vi "Digital_Bridge_3_kart.vi"() -> ()   [LabVIEW 2014] (continued)
            # "Bu bölüm, iterasyona (tekrarlamalı işleme) bağlı olarak Reserve ayarının maksimumda mı yoksa minimumda mı olacağını belirler. Aynı zamanda, ölçüm sürecinin başlangıcında kullanılacak olan sensitivity  değerleri de bu bölümde ayarlanır. Bu ayarlar, ölçüm sırasında cihazın hassasiyetini ve çalışma aralığını doğru şekilde belirlemek için gereklidir."
            # "ana denge"
            n1007 = case shown="True" "Ana denge Switch" {
              frame False {
              }
              frame True {
                # "Ana denge switch ayarlanıyor ve global x ve y set ediliyor"
                n1008 = flat-sequence {
                  frame #0 {
                    n1009 = local read "iterasyon AD"() -> (w4688:dbl)
                    n1010 = Equal?(x=w4688, y=0.0) -> (x = y?=w4689:bool)
                    n1011 = case shown="True" w4689 {
                      frame False {
                      }
                      frame True {
                        n1012 = local read "1 or 10"() -> (w4691:i32)
                        n1013 = case shown="1" w4691 {
                          frame 0, Default {
                          }
                          frame 1 {
                            n1014 = local write "iterasyon AD"(1.0 ("iterasyon WAGNER")) -> ()
                          }
                        }
                      }
                    }
                  }
                  frame #1 {
                    n1015 = local read "iterasyon AD"() -> (w4693:dbl)
                    n1016 = local read "1 or 10"() -> (w4697:i32)
                    n1017 = Equal?(x=w4697, y=1) -> (x = y?=w4698:bool)
                    n1018 = Greater?(x=w4693, y=0.0) -> (0:w4695:bool)
                    n1019 = Or(x=w4695, y=w4698) -> (x .or. y?=w4694:bool)
                    n1020 = case shown="True" w4694 {
                      frame False {
                        n1021 = local read "Reserve AD"() -> (w4701:u16)
                        n1022 = case shown="0, Default" w4701 {
                          tunnel: ["0" ("Reserve(MAX-MIN)") "1" ("Reserve(MAX-MIN)") "2" ("Reserve(MAX-MIN)")] -> w4700
                          frame 0, Default {
                          }
                          frame 1 {
                          }
                          frame 2 {
                          }
                        }
                        n1023 = local read "GPIB In"() -> (w4702:refnum<visa-resource-name>)
                        n1024 = call "Reserve.vi"("Reserve(MAX-MIN)"=w4700, "VISA resource name"=w4702) -> ()  [unwired: 8 in, 2 out]
                      }
                      frame True {
                        n1025 = local read "GPIB In"() -> (w4707:refnum<visa-resource-name>)
                        n1026 = call "Reserve.vi"("Reserve(MAX-MIN)"="2", "VISA resource name"=w4707) -> ()  [unwired: 8 in, 2 out]
                      }
                    }
                  }
                  frame #2 {
                    n1027 = Wait (ms)(milliseconds to wait=u32 500) -> ()  [unwired: 1 out]
                  }
                  frame #3 {
                    w4710 = u16 1 items=["Wagner", "Ground"] ("Switch")
                    w4711 = u16 1 items=["Open All", "Ana Denge", "10R", "1R"] ("Ring")
                    n1028 = call "mux1.vi"("Ring"=w4711) -> ("error out"=w4712:errorcluster)  [unwired: 9 in]
                    n1029 = property on="Tab Control" class="TabCtl (strict)"("Value"=T4."Ana Denge" ("Tab Control")) -> ()  [unwired: 2 in, 2 out]
                    n1030 = call "mux2.vi"("Switch"=w4710, "error in (no error)"=w4712) -> ()  [unwired: 6 in, 1 out]
                  }
                  frame #4 {
                    n1031 = Wait (ms)(milliseconds to wait=u32 1000) -> ()  [unwired: 1 out]
                  }
                  frame #5 {
                    n1032 = local read "1 or 10"() -> (w4717:i32)
                    n1033 = local read "İterasyon X"() -> (w4720:dbl)
                    n1034 = Equal?(x=w4717, y=1) -> (x = y?=w4716:bool)
                    n1035 = Greater?(x=w4720, y=0.0) -> (0:w4715:bool)
                    n1036 = Or(x=w4715, y=w4716) -> (x .or. y?=w4714:bool)
                    n1037 = case shown="False" w4714 {
                      frame False {
                        n1038 = local read "Y Range AD"() -> (w4721:dbl)
                        n1039 = local read "X Range AD"() -> (w4722:dbl)
                        n1040 = global write "show_sensitivity.vi" "show sensitivity (ana denge  x)"(w4722) -> ()
                        n1041 = global write "show_sensitivity.vi" "show sensitivity (ana denge  y)"(w4721) -> ()
                      }
                      frame True {
                        w4723 = 10.0 ("Max. Hassasiyet")
                        n1042 = global write "show_sensitivity.vi" "show sensitivity (ana denge  x)"(w4723) -> ()
                        n1043 = global write "show_sensitivity.vi" "show sensitivity (ana denge  y)"(w4723) -> ()
                      }
                    }
                  }
                  frame #6 {
                    n1044 = local write "Ana denge Switch"(FALSE ("wagner switch")) -> ()
                    n1045 = local write "Start AD X"(TRUE ("START WAGNER")) -> ()
                  }
                }
              }
            }
            n1046 = case shown="True" "Start AD X" {
              frame False {
              }
              frame True {
                n1047 = flat-sequence {
                  frame #0 {
                    w4665 = u16 0 items=["A", "A-B"] ("Input Source (0: A)")
                    n1048 = local read "frekans index"() -> (w4660:dbl)
                    n1049 = local read "Frekanslar"() -> (w4661:dbl[])
                    n1050 = local read "Direnc 1 - Direnc 2"() -> (w4662:u32)
                    n1051 = local read "AD F/P Array"() -> (w4663:dbl[][])
                    n1052 = Index Array(array=w4661, index=w4660) -> (element=w4659:dbl)
                    n1053 = call "get_phase_element.vi"("index r"=w4662, "hz"=w4659, "Array"=w4663) -> ("element"=w4655:dbl)  [unwired: 8 in]
                    n1054 = Number To Fractional String(number=w4655) -> (F-format string=w4658:string)  [unwired: 3 in]
                    n1055 = local read "GPIB In"() -> (w4664:refnum<visa-resource-name>)
                    n1056 = Search and Replace String(input string=w4658, search string=",", replace string="." ("replace string (\"\")")) -> (result string=w4654:string)  [unwired: 5 in, 3 out]
                    n1057 = call "reference phase.vi"("Reference Phase (0.000 degrees)"=w4654, "VISA resource name"=w4664) -> ("error out"=w4666:errorcluster, "VISA resource name out"=w4667:refnum<visa-resource-name>)  [unwired: 8 in]
                    n1058 = call "input source.vi"("error in (no error)"=w4666, "Input Source (0: A)"=w4665, "VISA resource name"=w4667) -> ()  [unwired: 7 in, 2 out]
                  }
                  frame #1 {
                    n1059 = local read "İterasyon X"() -> (w4678:dbl)
                    n1060 = local read "1 or 10"() -> (w4682:i32)
                    n1061 = local read "frekans index"() -> (w4676:dbl)
                    n1062 = local read "control hz array"() -> (w4673:dbl[][])
                    n1063 = Greater?(x=w4678, y=0.0) -> (0:w4679:bool)
                    n1064 = call "change2d.vi"("reset(default false)"=FALSE, "index (col)"=w4676, "index (row)"=2, "read/write(T/F)"=TRUE, "2D Array"=w4673) -> ("result count"=w4671:dbl)  [unwired: 5 in, 1 out]
                    n1065 = Equal?(x=w4682, y=1) -> (x = y?=w4680:bool)
                    n1066 = local read "set"() -> (w4670:u16)
                    n1067 = Or(x=w4679, y=w4680) -> (x .or. y?=w4672:bool)
                    n1068 = Equal?(x=w4671, y=w4670) -> (x = y?=w4669:bool)
                    n1069 = Or(x=w4672, y=w4669) -> (x .or. y?=w4668:bool)
                    n1070 = case shown="True" w4668 {
                      frame False {
                        n1071 = local write "auto phase AD"(TRUE ("auto phase 10R")) -> ()
                        n1072 = local write "Start AD X"(FALSE ("auto phase 10R")) -> ()
                      }
                      frame True {
                        n1073 = local write "Contiune AD"(TRUE) -> ()
                        n1074 = local write "Start AD X"(FALSE ("START WAGNER")) -> ()
                      }
                    }
                  }
                }
              }
            }
            n1075 = case shown="True" "RESET SENS X" {
              frame False {
              }
              frame True {
                n1076 = local read "count meas"() -> (w4779:u16)
                n1077 = local read "iterasyon AD"() -> (w4777:dbl)
                n1078 = Greater?(x=w4779, y=u16 8) -> (0:w4775:bool)
                n1079 = Greater?(x=w4777, y=5.0) -> (0:w4774:bool)
                n1080 = Or(x=w4775, y=w4774) -> (x .or. y?=w4773:bool)
                n1081 = case shown="True" w4773 {
                  frame False {
                    n1082 = flat-sequence {
                      frame #0 {
                        n1083 = global read "show_sensitivity.vi" "show sensitivity (ana denge  x)"() -> (w4780:dbl)
                        n1084 = local read "GPIB In"() -> (w4781:refnum<visa-resource-name>)
                        n1085 = call "get_sensitivity.vi"("input 1"=w4780, "SR850 GPIB In"=w4781) -> ()  [unwired: 8 in, 2 out]
                      }
                      frame #1 {
                        n1086 = Wait (ms)(milliseconds to wait=u32 500) -> ()  [unwired: 1 out]
                      }
                      frame #2 {
                        n1087 = local write "RESET SENS X"(FALSE ("RESET SENS X")) -> ()
                        n1088 = local write "START X"(TRUE ("START X 4")) -> ()
                      }
                    }
                  }
                  frame True {
                    n1089 = local read "iterasyon AD"() -> (w4786:dbl)
                    n1090 = Greater?(x=w4786, y=5.0) -> (0:w4785:bool)
                    n1091 = case shown="False" w4785 {
                      frame False {
                        n1092 = flat-sequence {
                          frame #0 {
                            n1093 = local write "count meas"(u16 9 ("count meas")) -> ()
                            n1094 = local write "RESET SENS X"(FALSE ("Start 10R X")) -> ()
                            n1095 = local write "İterasyon X"(0.0 ("İterasyon X")) -> ()
                          }
                          frame #1 {
                            n1096 = local write "reset values"(TRUE ("Start 10R X")) -> ()
                            n1097 = local write "error"(TRUE ("Start 10R X")) -> ()
                          }
                        }
                      }
                      frame True {
                        n1098 = flat-sequence {
                          frame #0 {
                            n1099 = local write "count meas"(u16 10 ("count meas")) -> ()
                            n1100 = local write "RESET SENS X"(FALSE ("Start 10R X")) -> ()
                            n1101 = local write "İterasyon X"(0.0 ("İterasyon X")) -> ()
                          }
                          frame #1 {
                            n1102 = local write "reset values"(TRUE ("Start 10R X")) -> ()
                            n1103 = local write "error"(TRUE ("Start 10R X")) -> ()
                          }
                        }
                      }
                    }
                  }
                }
              }
            }
            n1104 = case shown="True" "START X" {
              frame False {
              }
              frame True {
                n1105 = flat-sequence {
                  frame #0 {
                    n1106 = local read "AD X(k-1)"() -> (w4799:dbl)
                    n1107 = local read "AD Xk"() -> (w4798:dbl)
                    n1108 = local write "input 2 x [ana denge]"(w4799) -> ()
                    n1109 = local write "input 1 x [ana denge]"(w4798) -> ()
                    n1110 = global write "DB_Global_4_kart-Test.vi" "amplitude 2/0"(w4798) -> ()
                  }
                  frame #1 {
                    n1111 = Wait (ms)(milliseconds to wait=u32 500) -> ()  [unwired: 1 out]
                  }
                  frame #2 {
                    n1112 = local write "START X"(FALSE ("START X 4")) -> ()
                    n1113 = local write "X"(TRUE ("START X")) -> ()
                  }
                  frame #3 {
                  }
                }
              }
            }
            n1114 = case shown="True" "Optimum Range 1" {
              frame False {
              }
              frame True {
                n1115 = flat-sequence {
                  frame #0 {
                    n1116 = global read "show_sensitivity.vi" "show sensitivity (ana denge  x)"() -> (w4326:dbl)
                    n1117 = local read "GPIB In"() -> (w4327:refnum<visa-resource-name>)
                    n1118 = call "get_sensitivity.vi"("input 1"=w4326, "SR850 GPIB In"=w4327) -> ()  [unwired: 8 in, 2 out]
                  }
                  frame #1 {
                    n1119 = call "set optimum range.vi"("denge degeri"=1.0) -> ("ok"=w4328:bool)  [unwired: 14 in]
                    n1120 = case shown="True" w4328 {
                      frame False {
                      }
                      frame True {
                        n1121 = local write "Optimum Range 1"(FALSE ("Optimum Range 1")) -> ()
                        n1122 = local write "PASS ANA D"(TRUE ("PASS ANA D")) -> ()
                      }
                    }
                  }
                }
              }
            }
            n1123 = case shown="True" "Start AD Y" {
              frame False {
              }
              frame True {
                n1124 = flat-sequence {
                  frame #0 {
                    w4762 = u16 0 items=["A", "A-B"] ("Input Source (0: A)")
                    n1125 = local read "frekans index"() -> (w4756:dbl)
                    n1126 = local read "Frekanslar"() -> (w4757:dbl[])
                    n1127 = local read "Direnc 1 - Direnc 2"() -> (w4759:u32)
                    n1128 = local read "AD F/P Array"() -> (w4760:dbl[][])
                    n1129 = Index Array(array=w4757, index=w4756) -> (element=w4758:dbl)
                    n1130 = call "get_phase_element.vi"("index r"=w4759, "hz"=w4758, "Array"=w4760) -> ("element"=w4752:dbl)  [unwired: 8 in]
                    n1131 = Number To Fractional String(number=w4752) -> (F-format string=w4753:string)  [unwired: 3 in]
                    n1132 = local read "GPIB In"() -> (w4761:refnum<visa-resource-name>)
                    n1133 = Search and Replace String(input string=w4753, search string=",", replace string="." ("replace string (\"\")")) -> (result string=w4751:string)  [unwired: 5 in, 3 out]
                    n1134 = call "reference phase.vi"("Reference Phase (0.000 degrees)"=w4751, "VISA resource name"=w4761) -> ("error out"=w4763:errorcluster, "VISA resource name out"=w4764:refnum<visa-resource-name>)  [unwired: 8 in]
                    n1135 = call "input source.vi"("error in (no error)"=w4763, "Input Source (0: A)"=w4762, "VISA resource name"=w4764) -> ()  [unwired: 7 in, 2 out]
                  }
                  frame #1 {
                    n1136 = local write "Boolean"(FALSE ("Boolean 4")) -> ()
                    n1137 = local write "RESET SENS Y"(TRUE ("START X")) -> ()
                    n1138 = local write "Start AD Y"(FALSE ("START Y 6")) -> ()
                  }
                }
              }
            }
            n1139 = case shown="True" "RESET SENS Y" {
              frame False {
              }
              frame True {
                n1140 = local read "count meas"() -> (w4731:u16)
                n1141 = local read "iterasyon AD"() -> (w4730:dbl)
                n1142 = Greater?(x=w4731, y=u16 8) -> (0:w4728:bool)
                n1143 = Greater?(x=w4730, y=5.0) -> (0:w4727:bool)
                n1144 = Or(x=w4728, y=w4727) -> (x .or. y?=w4726:bool)
                n1145 = case shown="True" w4726 {
                  frame False {
                    n1146 = flat-sequence {
                      frame #0 {
                        n1147 = global read "show_sensitivity.vi" "show sensitivity (ana denge  y)"() -> (w4733:dbl)
                        n1148 = local read "GPIB In"() -> (w4734:refnum<visa-resource-name>)
                        n1149 = call "get_sensitivity.vi"("input 1"=w4733, "SR850 GPIB In"=w4734) -> ()  [unwired: 8 in, 2 out]
                      }
                      frame #1 {
                        n1150 = Wait (ms)(milliseconds to wait=u32 500) -> ()  [unwired: 1 out]
                      }
                      frame #2 {
                        n1151 = local write "RESET SENS Y"(FALSE ("RESET SENS X")) -> ()
                        n1152 = local write "START Y"(TRUE ("START X 4")) -> ()
                      }
                    }
                  }
                  frame True {
                    n1153 = local read "iterasyon AD"() -> (w4739:dbl)
                    n1154 = Greater?(x=w4739, y=5.0) -> (0:w4738:bool)
                    n1155 = case shown="False" w4738 {
                      frame False {
                        n1156 = flat-sequence {
                          frame #0 {
                            n1157 = local write "count meas"(u16 9 ("count meas")) -> ()
                            n1158 = local write "RESET SENS Y"(FALSE ("Start 10R X")) -> ()
                            n1159 = local write "İterasyon X"(0.0 ("İterasyon X")) -> ()
                          }
                          frame #1 {
                            n1160 = local write "reset values"(TRUE ("Start 10R X")) -> ()
                            n1161 = local write "error"(TRUE ("Start 10R X")) -> ()
                          }
                        }
                      }
                      frame True {
                        n1162 = flat-sequence {
                          frame #0 {
                            n1163 = local write "count meas"(u16 10 ("count meas")) -> ()
                            n1164 = local write "RESET SENS Y"(FALSE ("Start 10R X")) -> ()
                            n1165 = local write "İterasyon X"(0.0 ("İterasyon X")) -> ()
                          }
                          frame #1 {
                            n1166 = local write "reset values"(TRUE ("Start 10R X")) -> ()
                            n1167 = local write "error"(TRUE ("Start 10R X")) -> ()
                          }
                        }
                      }
                    }
                  }
                }
              }
            }
            n1168 = case shown="True" "START Y" {
              frame False {
              }
              frame True {
                n1169 = flat-sequence {
                  frame #0 {
                    n1170 = local read "AD Y(k-1)"() -> (w4769:dbl)
                    n1171 = local read "AD Yk"() -> (w4768:dbl)
                    n1172 = local write "input 1 y [ana denge]"(w4768) -> ()
                    n1173 = local write "input 2 y [ana denge]"(w4769) -> ()
                    n1174 = global write "DB_Global_4_kart-Test.vi" "phase 2/ 0"(w4768) -> ()
                  }
                  frame #1 {
                    n1175 = Wait (ms)(milliseconds to wait=u32 500) -> ()  [unwired: 1 out]
                  }
                  frame #2 {
                    n1176 = local write "START Y"(FALSE ("START X")) -> ()
                    n1177 = local write "Y"(TRUE ("START X")) -> ()
                  }
                }
              }
            }
            n1178 = case shown="True" "Contiune AD" {
              frame False {
              }
              frame True {
                n1179 = local read "1 or 10"() -> (w4384:i32)
                n1180 = local read "iterasyon AD"() -> (w4388:dbl)
                n1181 = local read "frekans index"() -> (w4377:dbl)
                n1182 = local read "control hz array"() -> (w4381:dbl[][])
                n1183 = case shown="1" w4384 {
                  tunnel: [FALSE TRUE] -> w4385
                  frame 10, Default {
                  }
                  frame 1 {
                  }
                }
                n1184 = call "change2d.vi"("reset(default false)"=FALSE, "index (col)"=w4377, "index (row)"=2, "read/write(T/F)"=TRUE, "2D Array"=w4381) -> ("result count"=w4382:dbl)  [unwired: 5 in, 1 out]
                n1185 = local read "set"() -> (w4383:u16)
                n1186 = Greater?(x=w4388, y=0.0) -> (0:w4386:bool)
                n1187 = Equal?(x=w4382, y=w4383) -> (x = y?=w4376:bool)
                n1188 = Or(x=w4386, y=w4385) -> (x .or. y?=w4375:bool)
                n1189 = Or(x=w4375, y=w4376) -> (x .or. y?=w4374:bool)
                n1190 = case shown="True" w4374 {
                  frame False {
                    n1191 = local write "Contiune AD"(FALSE ("START WAGNER")) -> ()
                    n1192 = local write "RESET SENS X"(TRUE ("START X")) -> ()
                    n1193 = local write "Boolean"(FALSE ("Boolean 4")) -> ()
                  }
                  frame True {
                    n1194 = local write "Optimum Range 1"(TRUE ("START X")) -> ()
                    n1195 = local write "Contiune AD"(FALSE ("Boolean 4")) -> ()
                    n1196 = local write "Boolean"(FALSE ("Boolean 4")) -> ()
                  }
                }
              }
            }
            n1197 = case shown="True" "PASS ANA D" {
              frame False {
              }
              frame True {
                n1198 = flat-sequence {
                  frame #0 {
                    n1199 = Wait (ms)(milliseconds to wait=u32 3000) -> ()  [unwired: 1 out]
                  }
                  frame #1 {
                    n1200 = local read "Output Denge Kosulu x2_y2"() -> (w4577:dbl[][])
                    n1201 = local read "Other Array"() -> (w4598:dbl[])
                    n1202 = for {
                      N: 7 -> [_]
                      shift-right: [w4631] -> w4601
                      shift-left: w4598 -> [w4634]
                      i -> [w4633]
                      n1203 = case shown="6" w4633 {
                        tunnel: [1.0 ("iterasyon WAGNER") w4636 w4637 w4638 w4639 w4640 w4641] -> w4632
                        frame 0, Default {
                        }
                        frame 1 {
                          n1204 = local read "Iterasyon Successful"() -> (w4636:dbl)
                        }
                        frame 2 {
                          n1205 = local read "Direnc 1 - Direnc 2"() -> (w4637:u32)
                        }
                        frame 3 {
                          n1206 = local read "olcum"() -> (w4638:u16)
                        }
                        frame 4 {
                          n1207 = local read "set"() -> (w4639:u16)
                        }
                        frame 5 {
                          n1208 = local read "frekans index"() -> (w4640:dbl)
                        }
                        frame 6 {
                          n1209 = local read "iterasyon AD"() -> (w4641:dbl)
                        }
                      }
                      n1210 = Replace Array Subset(array=w4634, new element=w4632, index=w4633) -> (w4631:dbl[])
                    }
                    n1211 = control-ref of="Default Values Listbox"() -> (w4581:refnum<vi>)
                    n1212 = local read "Output Denge Kosulu x1_x2"() -> (w4576:dbl[][])
                    n1213 = local read "Outpu Denge Kosulu y1_y2"() -> (w4575:dbl[][])
                    n1214 = local read "Frekanslar"() -> (w4562:dbl[])
                    n1215 = local read "Cluster"() -> (w4579:T2)
                    n1216 = local read "Cluster 2"() -> (w4578:T1)
                    n1217 = Array Size(array=w4562) -> (size(s)=w4561:i32)
                    n1218 = call "merge_x_y.vi"("frekans size"=w4561, "y1_y2"=w4575, "x1_x2"=w4576) -> ("x1_x2_y1_y2"=w4574:dbl[][])  [unwired: 8 in]
                    n1219 = local read "input values"() -> (w4580:dbl[])
                    n1220 = local read "default values"() -> (w4602:T3)
                    n1221 = local read "Sheet name"() -> (w4599:string)
                    n1222 = local read "Other Boolean Array"() -> (w4597:bool[])
                    n1223 = for {
                      N: 5 -> [_]
                      shift-right: [w4622] -> w4600
                      shift-left: w4597 -> [w4625]
                      i -> [w4624]
                      n1224 = case shown="2" w4624 {
                        tunnel: [FALSE FALSE FALSE FALSE FALSE] -> w4623
                        frame 0, Default {
                        }
                        frame 1 {
                        }
                        frame 2 {
                        }
                        frame 3 {
                        }
                        frame 4 {
                        }
                      }
                      n1225 = Replace Array Subset(array=w4625, new element=w4623, index=w4624) -> (w4622:bool[])
                    }
                    n1226 = call "Pass.vi"("Other Array"=w4601, "Other Boolean Array"=w4600, "Denge Kosulu x2_y2"=w4577, "LstBox Refnum"=w4581, "Cluster"=w4579, "F/P Array Cluster"=w4578, "Sheet name"=w4599, "default values"=w4602, "x1_x2_y1_y2"=w4574, "input values"=w4580) -> ("output values"=w4573:dbl[], "Output Other Boolean Array"=w4594:bool[], "Output Cluster"=w4572:T2, "Output F/P Array Cluster"=w4568:T1, "output default values"=w4596:T11, "Output Iterasyon Successful"=w4595:dbl, "Denge Seçimi"=w4583:u8, "end time"=w4582:string)  [unwired: 1 in, 1 out]
                    n1227 = local write "input values"(w4573) -> ()
                    n1228 = Unbundle By Name(w4572) -> ("F Values Array"=w4571:dbl[][], "control hz array"=w4570:dbl[][], "extra default values"=w4569:dbl[][])
                    n1229 = Unbundle By Name(w4568) -> ("AD F/P Array"=w4567:dbl[][], "10R F/P Array"=w4566:dbl[][], "1R F/P Array"=w4565:dbl[][], "Wagner F/P Array"=w4564:dbl[][], "Kelvin F/P Array"=w4563:dbl[][])
                    n1230 = local write "default values"(w4596) -> ()
                    n1231 = local write "Iterasyon Successful"(w4595) -> ()
                    n1232 = local write "AD F/P Array"(w4567) -> ()
                    n1233 = local write "10R F/P Array"(w4566) -> ()
                    n1234 = local write "1R F/P Array"(w4565) -> ()
                    n1235 = local write "Wagner F/P Array"(w4564) -> ()
                    n1236 = local write "Kelvin F/P Array"(w4563) -> ()
                    n1237 = local write "F Values Array"(w4571) -> ()
                    n1238 = local write "control hz array"(w4570) -> ()
                    n1239 = local write "extra default values"(w4569) -> ()
                    n1240 = Index Array(array=w4594, index #1=0 ("index"), index #2=1 ("index"), index #3=2 ("index"), index #4=3 ("index"), index #5=4 ("index")) -> (element #1=w4588:bool, element #2=w4587:bool, element #3=w4586:bool, element #4=w4585:bool, element #5=w4584:bool)
                    n1241 = case shown="True" w4588 {
                      frame False {
                      }
                      frame True {
                        n1242 = local write "PASS ANA D"(FALSE ("PASS ANA D")) -> ()
                        n1243 = local write "reset values"(TRUE ("reset values")) -> ()
                        n1244 = local write "pass hz"(TRUE ("pass hz")) -> ()
                        n1245 = local write "Boolean"(TRUE ("Boolean 4")) -> ()
                      }
                    }
                    n1246 = case shown="True" w4587 {
                      tunnel: w4583 -> [_ w4616]
                      frame False {
                      }
                      frame True {
                        n1247 = local write "wagner switch"(TRUE ("10R switch")) -> ()
                        n1248 = local write "PASS ANA D"(FALSE ("PASS ANA D")) -> ()
                        n1249 = local write "count meas"(u16 0 ("count meas")) -> ()
                        n1250 = local write "Denge Seçimi"(w4616) -> ()
                        n1251 = local write "Boolean"(TRUE ("Boolean 4")) -> ()
                      }
                    }
                    n1252 = case shown="True" w4586 {
                      tunnel: w4582 -> [_ w4611]
                      frame False {
                      }
                      frame True {
                        n1253 = local write "PASS ANA D"(FALSE ("PASS ANA D")) -> ()
                        n1254 = local write "reset values"(TRUE ("reset values")) -> ()
                        n1255 = local write "end time"(w4611) -> ()
                        n1256 = local write "Boolean"(TRUE ("Boolean 4")) -> ()
                      }
                    }
                    n1257 = case shown="True" w4585 {
                      frame False {
                      }
                      frame True {
                        n1258 = local write "RESET SENS X"(TRUE ("RESET SENS X 4")) -> ()
                        n1259 = local write "PASS ANA D"(FALSE ("PASS ANA D")) -> ()
                      }
                    }
                    n1260 = case shown="True" w4584 {
                      frame False {
                      }
                      frame True {
                        n1261 = local write "RESET SENS Y"(TRUE ("RESET SENS Y 4")) -> ()
                        n1262 = local write "PASS ANA D"(FALSE ("PASS ANA D")) -> ()
                      }
                    }
                  }
                  frame #2 {
                  }
                }
              }
            }
            n1263 = case shown="True" "auto phase AD" {
              frame False {
              }
              frame True {
                n1264 = flat-sequence {
                  frame #0 {
                    n1265 = local read "GPIB In"() -> (w4645:refnum<visa-resource-name>)
                    n1266 = local read "GPIB In"() -> (w4643:refnum<visa-resource-name>)
                    n1267 = call "Reserve.vi"("Reserve(MAX-MIN)"="2", "VISA resource name"=w4643) -> ()  [unwired: 8 in, 2 out]
                    n1268 = call "reference phase.vi"("Reference Phase (0.000 degrees)"="0", "VISA resource name"=w4645) -> ()  [unwired: 8 in, 2 out]
                  }
                  frame #1 {
                    w4647 = u16 0 items=["100 nV", "200 nV", "500 nV", "1 uV", "2 uV", "5 uV", "10 uV", "20 uV", "50 uV", "100 uV", "200 uV", "500 uV", "1 mV"] ("Min. Hassasiyet")
                    n1269 = local read "X Range AD"() -> (w4646:dbl)
                    n1270 = local read "GPIB In"() -> (w4648:refnum<visa-resource-name>)
                    n1271 = call "GAIN BASIC.vi"("SR850 GPIB In"=w4648, "Max. Hassasiyet"=w4646, "Auto Gain (False)"=FALSE, "Min. Hassasiyet"=w4647) -> ()  [unwired: 10 in, 2 out]
                  }
                  frame #2 {
                    n1272 = local read "X 1.input AD"() -> (w4650:dbl)
                    n1273 = global write "DB_Global_4_kart-Test.vi" "phase 2/ 0"(w4650) -> ()
                    n1274 = global write "DB_Global_4_kart-Test.vi" "amplitude 2/0"(w4650) -> ()
                  }
                  frame #3 {
                    n1275 = Wait (ms)(milliseconds to wait=u32 750) -> ()  [unwired: 1 out]
                  }
                  frame #4 {
                    n1276 = local write "read x1 y1"(TRUE ("output x")) -> ()
                    n1277 = local write "auto phase AD"(FALSE ("auto phase wagner")) -> ()
                  }
                }
              }
            }
            n1278 = case shown="True" "read x1 y1" {
              frame False {
              }
              frame True {
                n1279 = local read "X Range AD"() -> (w4310:dbl)
                n1280 = call "only_x_and_y_output.vi"("range"=w4310) -> ("cycle 2"=w4314:bool, "range 2"=w4311:dbl, "Output Y"=w4312:dbl, "Output X"=w4313:dbl)  [unwired: 7 in]
                n1281 = case shown="False" w4314 {
                  tunnel: w4313 -> [w4317 _]
                  tunnel: w4312 -> [w4316 _]
                  tunnel: w4311 -> [w4315 w4325]
                  frame False {
                    n1282 = flat-sequence {
                      tunnel: w4317 -> [w4320]
                      tunnel: w4316 -> [w4319]
                      tunnel: w4315 -> [w4318]
                      frame #0 {
                        n1283 = local write "X Range AD"(w4318) -> ()
                        n1284 = local write "Output Y1"(w4319) -> ()
                        n1285 = local write "Output X1"(w4320) -> ()
                      }
                      frame #1 {
                        n1286 = local read "X 2.input AD"() -> (w4321:dbl)
                        n1287 = global write "DB_Global_4_kart-Test.vi" "amplitude 2/0"(w4321) -> ()
                      }
                      frame #2 {
                        n1288 = Wait (ms)(milliseconds to wait=u32 750) -> ()  [unwired: 1 out]
                      }
                      frame #3 {
                        n1289 = local write "read x2 y2"(TRUE ("output x")) -> ()
                        n1290 = local write "read x1 y1"(FALSE ("output x")) -> ()
                      }
                    }
                  }
                  frame True {
                    n1291 = local write "X Range AD"(w4325) -> ()
                  }
                }
              }
            }
            n1292 = case shown="True" "RANGE KONTROL Y" {
              frame False {
              }
              frame True {
                n1293 = local read "Outpu Denge Kosulu y1_y2"() -> (w4436:dbl[][])
                n1294 = local read "input 1 y [ana denge]"() -> (w4437:dbl)
                n1295 = local read "input 2 y [ana denge]"() -> (w4438:dbl)
                n1296 = local read "output 2 y [ana denge]"() -> (w4432:dbl)
                n1297 = local read "frekans index"() -> (w4429:dbl)
                n1298 = local read "iterasyon AD"() -> (w4435:dbl)
                n1299 = local read "output 1 y [ana denge]"() -> (w4434:dbl)
                n1300 = call "Range Kontrol Y.vi"("denge degeri"=1.0, "iterasyon Denge"=w4435, "frekans index"=w4429, "Denge Kosulu y1_y2"=w4436, "Yk"=w4437, "Y(k-1)"=w4438, "output y 1"=w4434, "output y 2"=w4432) -> ("Output Y(k-1)"=w4428:dbl, "result output y"=w4439:dbl, "KONTROL X"=w4431:bool, "IF ELSE"=w4430:bool)  [unwired: 8 in]
                n1301 = local write "AD Y(k-1)"(w4428) -> ()
                n1302 = local write "result output y [AD]"(w4439) -> ()
                n1303 = flat-sequence {
                  tunnel: w4431 -> [w4441]
                  tunnel: w4430 -> [w4440]
                  frame #0 {
                    n1304 = case shown="True" w4440 {
                      frame False {
                      }
                      frame True {
                        n1305 = local write "IF ELSE Y"(TRUE ("IF ELSE X 4")) -> ()
                      }
                    }
                    n1306 = case shown="True" w4441 {
                      frame False {
                      }
                      frame True {
                        n1307 = local write "KONTROL X"(TRUE ("KONTROL Y 4")) -> ()
                      }
                    }
                  }
                  frame #1 {
                    n1308 = local write "RANGE KONTROL Y"(FALSE ("KONTROL Y 4")) -> ()
                    n1309 = local read "İterasyon Y"() -> (w4445:dbl)
                    n1310 = Increment(x=w4445) -> (x+1=w4444:dbl)
                    n1311 = local write "İterasyon Y"(w4444) -> ()
                  }
                }
              }
            }
            n1312 = case shown="True" "RANGE KONTROL X" {
              frame False {
              }
              frame True {
                n1313 = local read "Output Denge Kosulu x1_x2"() -> (w4517:dbl[][])
                n1314 = local read "input 1 x [ana denge]"() -> (w4518:dbl)
                n1315 = local read "input 2 x [ana denge]"() -> (w4519:dbl)
                n1316 = local read "output 2 x [ana denge]"() -> (w4513:dbl)
                n1317 = local read "frekans index"() -> (w4509:dbl)
                n1318 = local read "iterasyon AD"() -> (w4516:dbl)
                n1319 = local read "output 1 x [ana denge]"() -> (w4515:dbl)
                n1320 = call "Range Kontrol X.vi"("denge degeri"=1.0, "iterasyon Denge"=w4516, "frekans index"=w4509, "Denge Kosulu x1_x2"=w4517, "Xk"=w4518, "X(k-1)"=w4519, "output x 1"=w4515, "output x 2"=w4513) -> ("Output X(k-1)"=w4508:dbl, "result output x"=w4520:dbl, "KONTROL Y"=w4512:bool, "IF ELSE"=w4511:bool, "Start Denge Y"=w4510:bool)  [unwired: 7 in]
                n1321 = local write "AD X(k-1)"(w4508) -> ()
                n1322 = local write "result output x [AD]"(w4520) -> ()
                n1323 = flat-sequence {
                  tunnel: w4512 -> [w4523]
                  tunnel: w4511 -> [w4522]
                  tunnel: w4510 -> [w4521]
                  frame #0 {
                    n1324 = case shown="True" w4521 {
                      frame False {
                      }
                      frame True {
                        n1325 = local write "Start AD Y"(TRUE ("Start Wagner Y")) -> ()
                      }
                    }
                    n1326 = case shown="True" w4522 {
                      frame False {
                      }
                      frame True {
                        n1327 = local write "IF ELSE X"(TRUE ("IF ELSE X 4")) -> ()
                      }
                    }
                    n1328 = case shown="True" w4523 {
                      frame False {
                      }
                      frame True {
                        n1329 = local write "KONTROL Y"(TRUE ("KONTROL Y 4")) -> ()
                      }
                    }
                  }
                  frame #1 {
                    n1330 = local write "RANGE KONTROL X"(FALSE ("KONTROL Y 4")) -> ()
                    n1331 = local read "İterasyon X"() -> (w4527:dbl)
                    n1332 = Increment(x=w4527) -> (x+1=w4528:dbl)
                    n1333 = local write "İterasyon X"(w4528) -> ()
                  }
                }
              }
            }
            n1334 = case shown="True" "Y" {
              frame False {
              }
              frame True {
                n1335 = local read "İterasyon Y"() -> (w4468:dbl)
                n1336 = local read "AD Y(k-1)"() -> (w4469:dbl)
                n1337 = call "Y.vi"("Y(k-1)"=w4469, "İterasyon Denge"=w4468, "denge degeri"=1.0) -> ("error"=w4466:bool, "output Y(k-1)"=w4463:dbl, "output y 1"=w4464:dbl, "cycle"=w4465:bool)  [unwired: 5 in]
                n1338 = case shown="False" w4465 {
                  tunnel: w4466 -> [w4472 _]
                  tunnel: w4464 -> [w4471 _]
                  tunnel: w4463 -> [w4470 _]
                  frame False {
                    n1339 = case shown="True" w4472 {
                      frame False {
                        n1340 = local write "Y1"(TRUE ("X1 4")) -> ()
                        n1341 = local write "Y"(FALSE ("X 4")) -> ()
                      }
                      frame True {
                        n1342 = local write "error"(TRUE ("X1 4")) -> ()
                        n1343 = local write "Y"(FALSE ("X 4")) -> ()
                      }
                    }
                    n1344 = local write "output 1 y [ana denge]"(w4471) -> ()
                    n1345 = local write "input 2 y [ana denge]"(w4470) -> ()
                    n1346 = local write "AD Y(k-1)"(w4470) -> ()
                  }
                  frame True {
                  }
                }
              }
            }
            n1347 = case shown="True" "X" {
              frame False {
              }
              frame True {
                n1348 = local read "İterasyon X"() -> (w4551:dbl)
                n1349 = local read "AD X(k-1)"() -> (w4552:dbl)
                n1350 = call "X.vi"("X(k-1)"=w4552, "İterasyon Denge"=w4551, "denge degeri"=1.0) -> ("error"=w4549:bool, "output X(k-1)"=w4546:dbl, "output x 1"=w4547:dbl, "cycle"=w4548:bool)  [unwired: 5 in]
                n1351 = case shown="False" w4548 {
                  tunnel: w4549 -> [w4555 _]
                  tunnel: w4547 -> [w4554 _]
                  tunnel: w4546 -> [w4553 _]
                  frame False {
                    n1352 = local write "output 1 x [ana denge]"(w4554) -> ()
                    n1353 = case shown="True" w4555 {
                      frame False {
                        n1354 = local write "X1"(TRUE ("X1 4")) -> ()
                        n1355 = local write "X"(FALSE ("X 4")) -> ()
                      }
                      frame True {
                        n1356 = local write "error"(TRUE ("X1 4")) -> ()
                        n1357 = local write "X"(FALSE ("X 4")) -> ()
                      }
                    }
                    n1358 = local write "AD X(k-1)"(w4553) -> ()
                    n1359 = local write "input 2 x [ana denge]"(w4553) -> ()
                  }
                  frame True {
                  }
                }
              }
            }
            n1360 = case shown="True" "read x2 y2" {
              frame False {
              }
              frame True {
                n1361 = local read "X Range AD"() -> (w4294:dbl)
                n1362 = call "only_x_and_y_output.vi"("range"=w4294) -> ("cycle 2"=w4298:bool, "range 2"=w4295:dbl, "Output Y"=w4296:dbl, "Output X"=w4297:dbl)  [unwired: 7 in]
                n1363 = case shown="False" w4298 {
                  tunnel: w4297 -> [w4301 _]
                  tunnel: w4296 -> [w4300 _]
                  tunnel: w4295 -> [w4299 w4309]
                  frame False {
                    n1364 = flat-sequence {
                      tunnel: w4301 -> [w4304]
                      tunnel: w4300 -> [w4303]
                      tunnel: w4299 -> [w4302]
                      frame #0 {
                        n1365 = local write "Output X2"(w4304) -> ()
                        n1366 = local write "Output Y2"(w4303) -> ()
                        n1367 = local write "X Range AD"(w4302) -> ()
                      }
                      frame #1 {
                        n1368 = global write "DB_Global_4_kart-Test.vi" "amplitude 2/0"(0.0) -> ()
                      }
                      frame #2 {
                        n1369 = Wait (ms)(milliseconds to wait=u32 750) -> ()  [unwired: 1 out]
                      }
                      frame #3 {
                        n1370 = local write "result phase"(TRUE ("result phase 4")) -> ()
                        n1371 = local write "read x2 y2"(FALSE ("output y")) -> ()
                      }
                    }
                  }
                  frame True {
                    n1372 = local write "X Range AD"(w4309) -> ()
                  }
                }
              }
            }
            n1373 = case shown="True" "Y1" {
              frame False {
              }
              frame True {
                n1374 = local read "output 1 y [ana denge]"() -> (w4455:dbl)
                n1375 = local read "İterasyon Y"() -> (w4452:dbl)
                n1376 = local read "AD Y(k-1)"() -> (w4454:dbl)
                n1377 = local read "AD Yk"() -> (w4453:dbl)
                n1378 = call "Y1.vi"("denge degeri"=1.0, "İterasyon Denge"=w4452, "Yk"=w4453, "Y(k-1)"=w4454, "output y 1"=w4455) -> ("Output Yk"=w4448:dbl, "output y 2"=w4447:dbl, "cycle"=w4449:bool, "error"=w4450:bool)  [unwired: 7 in]
                n1379 = case shown="False" w4449 {
                  tunnel: w4450 -> [w4458 _]
                  tunnel: w4448 -> [w4457 _]
                  tunnel: w4447 -> [w4456 _]
                  frame False {
                    n1380 = case shown="False" w4458 {
                      frame False {
                        n1381 = local write "RANGE KONTROL Y"(TRUE ("RANGE KONTROL X 4")) -> ()
                        n1382 = local write "Y1"(FALSE ("X1 4")) -> ()
                      }
                      frame True {
                        n1383 = local write "error"(TRUE ("X1 4")) -> ()
                        n1384 = local write "Y1"(FALSE ("X1 4")) -> ()
                      }
                    }
                    n1385 = local write "output 2 y [ana denge]"(w4456) -> ()
                    n1386 = local write "AD Yk"(w4457) -> ()
                  }
                  frame True {
                  }
                }
              }
            }
            n1387 = case shown="True" "IF ELSE Y" {
              frame False {
              }
              frame True {
                n1388 = local read "input 1 y [ana denge]"() -> (w4417:dbl)
                n1389 = local read "input 2 y [ana denge]"() -> (w4418:dbl)
                n1390 = local read "output 1 y [ana denge]"() -> (w4421:dbl)
                n1391 = local read "output 2 y [ana denge]"() -> (w4422:dbl)
                n1392 = local read "result output y [AD]"() -> (w4423:dbl)
                n1393 = call "If Else Y.vi"("denge degeri"=1.0, "Yk"=w4417, "Y(k-1)"=w4418, "output y 1"=w4421, "output y 2"=w4422, "result output y"=w4423) -> ("Output Y(k-1)"=w4416:dbl, "Start Y"=w4419:bool)  [unwired: 8 in]
                n1394 = local write "AD Y(k-1)"(w4416) -> ()
                n1395 = case shown="True" w4419 {
                  frame False {
                  }
                  frame True {
                    n1396 = local read "count meas"() -> (w4424:u16)
                    n1397 = local write "RESET SENS Y"(TRUE ("START X 4")) -> ()
                    n1398 = Increment(x=w4424) -> (x+1=w4425:u16)
                    n1399 = local write "count meas"(w4425) -> ()
                    n1400 = local write "IF ELSE Y"(FALSE ("IF ELSE X 4")) -> ()
                  }
                }
              }
            }
            n1401 = case shown="True" "X1" {
              frame False {
              }
              frame True {
                n1402 = local read "output 1 x [ana denge]"() -> (w4538:dbl)
                n1403 = local read "İterasyon X"() -> (w4535:dbl)
                n1404 = local read "AD X(k-1)"() -> (w4537:dbl)
                n1405 = local read "AD Xk"() -> (w4536:dbl)
                n1406 = call "X1.vi"("denge degeri"=1.0, "İterasyon Denge"=w4535, "Xk"=w4536, "X(k-1)"=w4537, "output x 1"=w4538) -> ("Output Xk"=w4531:dbl, "output x 2"=w4530:dbl, "cycle"=w4532:bool, "error"=w4533:bool)  [unwired: 7 in]
                n1407 = case shown="False" w4532 {
                  tunnel: w4533 -> [w4541 _]
                  tunnel: w4531 -> [w4540 _]
                  tunnel: w4530 -> [w4539 _]
                  frame False {
                    n1408 = case shown="True" w4541 {
                      frame False {
                        n1409 = local write "RANGE KONTROL X"(TRUE ("RANGE KONTROL X 4")) -> ()
                        n1410 = local write "X1"(FALSE ("X1 4")) -> ()
                      }
                      frame True {
                        n1411 = local write "error"(TRUE ("X1 4")) -> ()
                        n1412 = local write "X1"(FALSE ("X1 4")) -> ()
                      }
                    }
                    n1413 = local write "output 2 x [ana denge]"(w4539) -> ()
                    n1414 = local write "AD Xk"(w4540) -> ()
                  }
                  frame True {
                  }
                }
              }
            }
            n1415 = case shown="True" "IF ELSE X" {
              frame False {
              }
              frame True {
                n1416 = local read "input 1 x [ana denge]"() -> (w4497:dbl)
                n1417 = local read "output 1 x [ana denge]"() -> (w4501:dbl)
                n1418 = local read "output 2 x [ana denge]"() -> (w4502:dbl)
                n1419 = local read "input 2 x [ana denge]"() -> (w4498:dbl)
                n1420 = local read "result output x [AD]"() -> (w4503:dbl)
                n1421 = call "If Else X.vi"("denge degeri"=1.0, "Xk"=w4497, "X(k-1)"=w4498, "output x 1"=w4501, "output x 2"=w4502, "result output x"=w4503) -> ("Output X(k-1)"=w4496:dbl, "Start X"=w4499:bool)  [unwired: 8 in]
                n1422 = local write "AD X(k-1)"(w4496) -> ()
                n1423 = case shown="True" w4499 {
                  frame False {
                  }
                  frame True {
                    n1424 = local read "count meas"() -> (w4504:u16)
                    n1425 = local write "RESET SENS X"(TRUE ("START X 4")) -> ()
                    n1426 = local write "IF ELSE X"(FALSE ("IF ELSE X 4")) -> ()
                    n1427 = Increment(x=w4504) -> (x+1=w4505:u16)
                    n1428 = local write "count meas"(w4505) -> ()
                  }
                }
              }
            }
            n1429 = case shown="True" "result phase" {
              frame False {
              }
              frame True {
                n1430 = flat-sequence {
                  tunnel: [w4339] -> w4334
                  tunnel: w4334 -> [w4355]
                  tunnel: [w4355] -> w4333
                  tunnel: w4333 -> [w4360]
                  tunnel: [w4360] -> w4332
                  tunnel: w4332 -> [w4366]
                  frame #0 {
                    # "pi"
                    n1431 = local read "Output X1"() -> (w4338:dbl)
                    n1432 = local read "Output X2"() -> (w4337:dbl)
                    n1433 = local read "Output Y1"() -> (w4336:dbl)
                    n1434 = local read "Output Y2"() -> (w4335:dbl)
                    n1435 = local read "GPIB In"() -> (w4344:refnum<visa-resource-name>)
                    n1436 = call "return phase.vi"("VISA resource name"=w4344) -> ("return phase"=w4340:string)  [unwired: 10 in]
                    n1437 = Fract/Exp String To Number(use system decimal point (T)=FALSE, string=w4340) -> (number=w4342:dbl)  [unwired: 2 in, 1 out]
                    n1438 = formula code="theta = atan((y2-y1)/(x2-x1))*(180/pi)+phase;"("x1"=w4338, "x2"=w4337, "y1"=w4336, "y2"=w4335, "phase"=w4342, "pi"=3.141592653589793) -> ("theta"=w4339:dbl)
                  }
                  frame #1 {
                    n1439 = local read "frekans index"() -> (w4352:dbl)
                    n1440 = local read "Frekanslar"() -> (w4353:dbl[])
                    n1441 = local read "Direnc 1 - Direnc 2"() -> (w4357:u32)
                    n1442 = property on="Default Values Listbox" class="LstBox (strict)"() -> ("Item Names"=w4354:string[])  [unwired: 2 in, 2 out]
                    n1443 = Fract/Exp String To Number(string=w4354) -> (number=w4351:dbl[])  [unwired: 3 in, 1 out]
                    n1444 = local read "Cluster 2"() -> (w4347:T1)
                    n1445 = Index Array(array=w4353, index=w4352) -> (element=w4349:dbl)
                    n1446 = local read "AD F/P Array"() -> (w4358:dbl[][])
                    n1447 = Increment(x=w4357) -> (x+1=w4356:u32)
                    n1448 = Search 1D Array(1D array=w4351, element=w4349, start index (0)=0) -> (index of element=w4348:i32)
                    n1449 = Replace Array Subset(array=w4358, new element=w4355, index (row)=w4356, index (col)=w4348) -> (w4345:dbl[][])
                    n1450 = local write "AD F/P Array"(w4345) -> ()
                    n1451 = Bundle By Name(cluster=w4347, "AD F/P Array"=w4345) -> (w4346:T1)
                    n1452 = local write "Cluster 2"(w4346) -> ()
                  }
                  frame #2 {
                    n1453 = Wait (ms)(milliseconds to wait=u32 250) -> ()  [unwired: 1 out]
                  }
                  frame #3 {
                    w4363 = u16 0 items=["A", "A-B"] ("Input Source (0: A)")
                    n1454 = local read "GPIB In"() -> (w4362:refnum<visa-resource-name>)
                    n1455 = Number To Fractional String(number=w4366) -> (F-format string=w4367:string)  [unwired: 3 in]
                    n1456 = Search and Replace String(input string=w4367, search string=",", replace string="." ("replace string (\"\")")) -> (result string=w4361:string)  [unwired: 5 in, 3 out]
                    n1457 = call "reference phase.vi"("Reference Phase (0.000 degrees)"=w4361, "VISA resource name"=w4362) -> ("error out"=w4364:errorcluster, "VISA resource name out"=w4365:refnum<visa-resource-name>)  [unwired: 8 in]
                    n1458 = call "input source.vi"("error in (no error)"=w4364, "Input Source (0: A)"=w4363, "VISA resource name"=w4365) -> ()  [unwired: 7 in, 2 out]
                  }
                  frame #4 {
                    n1459 = local read "GPIB In"() -> (w4371:refnum<visa-resource-name>)
                    n1460 = local write "Contiune AD"(TRUE ("Contiune Wagner")) -> ()
                    n1461 = local write "result phase"(FALSE ("result phase 4")) -> ()
                    n1462 = call "Reserve.vi"("Reserve(MAX-MIN)"="0", "VISA resource name"=w4371) -> ()  [unwired: 8 in, 2 out]
                  }
                }
              }
            }
            n1463 = case shown="True" "KONTROL X" {
              frame False {
              }
              frame True {
                n1464 = local read "Output Denge Kosulu x1_x2"() -> (w4399:dbl[][])
                n1465 = local read "iterasyon AD"() -> (w4397:dbl)
                n1466 = local read "Manuel/Otomatik"() -> (w4405:enum16{"Manuel", "Otomatik"})
                n1467 = local read "frekans index"() -> (w4398:dbl)
